vi "Scale.vi"(8 "error in":errorcluster, 11 "Gen Refnum":refnum<vi>) -> (0 "error out":errorcluster, 3 "Scale out":refnum<class "Scale.lvclass">)   [LabVIEW 2014, in "Scale.lvclass"]
uses:
  Scale.lvclass
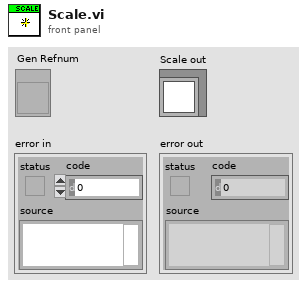
[diagram p1: front panel]
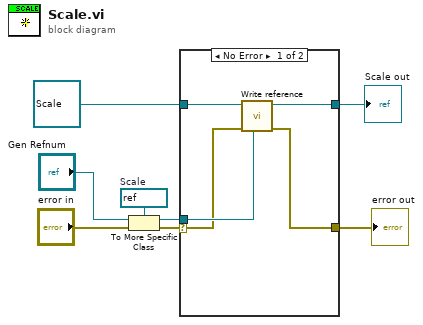
[diagram p0: block diagram]
diagram:
  w6 = refnum<vi> refnum  # Scale
  n1 = To More Specific Class(target class=w6, reference="Gen Refnum", error in="error in") -> (specific class reference=w4:refnum<vi>, error out=w5:errorcluster)
  n2 = case shown="No Error" w5 {
    selector: w5 -> [w11 w15]
    tunnel: w4 -> [w12 _]
    tunnel: refnum<class "Scale.lvclass"> refnum ("Scale in") -> [w13 w14]
    tunnel: [w9 w15] -> w1
    tunnel: [w10 w14] -> w2
    frame No Error {
      n3 = call-dynamic "Write reference.vi"("reference"=w12, "error in"=w11, "GObject in"=w13) -> ("error out"=w9:errorcluster, "GObject out"=w10:refnum<class "Scale.lvclass">)  [unwired: 5 in]
    }
    frame Error {
    }
  }
  "error out" <- w1
  "Scale out" <- w2
